vi "remote_I(t)-T at fixed V (V recorded), Ver. 2.vi"() -> ()   [LabVIEW 2014]
uses:
  C:/Program Files (x86)/National Instruments/LabVIEW 2014/examples/Instrument IO/Serial/support/Serial - Settings.ctl
  <vilib>/Instr/_visa.llb/VISA Configure Serial Port (Instr).vi
panel:
  out "Start":bool
  in  "获取的数据的字节最大值":u32=1000
  in  "终止符":u8=10 format="%.0x"
  in  "COM":refnum<visa-resource-name>="COM5"
  in  "串口设置":T1={"波特率"=38400, "数据比特"=8, "奇偶"=enum."None", "停止位"=10, "流控制"=0} {"流控制" items=["无"=0, "XON/XOFF"=1, "RTS/CTS"=2, "DTR/DSR"=4]; "停止位" items=["1.0"=10, "1.5"=15, "2.0"=20]; "数据比特" min=5 max=8 step=1; "波特率" items=["75"=75, "110"=110, "134"=134, "150"=150, "300"=300, "600"=600, "1200"=1200, "1800"=1800, "2400"=2400, "4800"=4800, "7200"=7200, "9600"=9600, "14400"=14400, "19200"=19200, "28800"=28800, "38400"=38400, "56000"=56000, "57600"=57600, "115200"=115200, "128000"=128000, "230400"=230400]}
  in  "终止符时结束读取？":bool=TRUE
  in  "Compliance":sgl=50.0
  in  "Start":bool
  out "File Path":path
  in  "Negative t":u32
  in  "Positive t":u32
  in  "Negative V":dbl min=-3.0 max=0.0
  in  "Positive V":dbl min=0.0 max=5.0 format="%#_3g"
  out "XY Graph":cluster{dbl[], dbl[]}[](graph)
  # "s"
  # "s"
  # "mA"
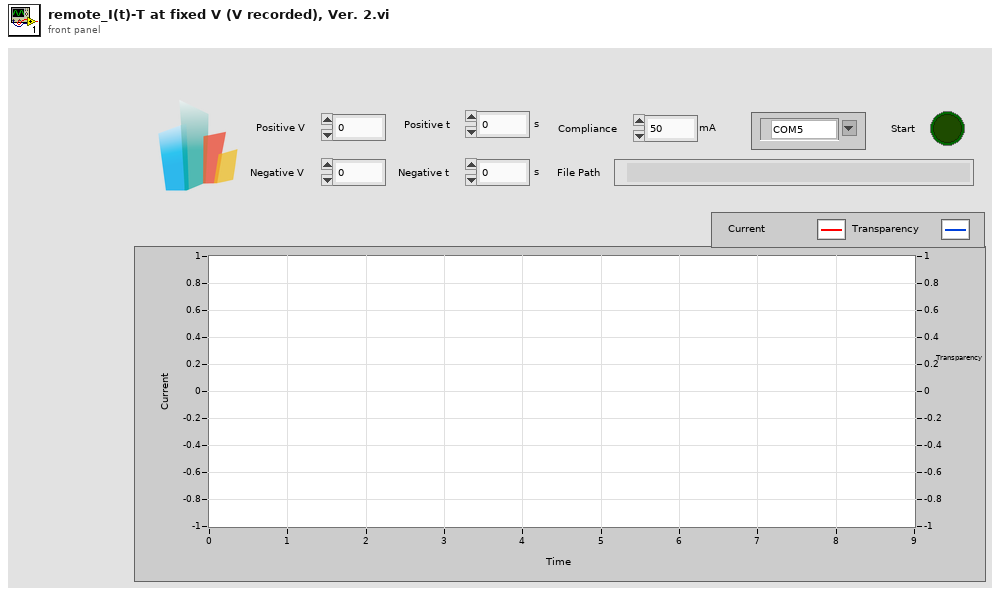
[diagram p1: front panel]
types:
  T1 = typedef "Serial - Settings.ctl" = cluster{"波特率":u32, "数据比特":u16, "奇偶":enum16{"None", "Odd", "Even", "Mark", "Space"}, "停止位":u16, "流控制":u16}
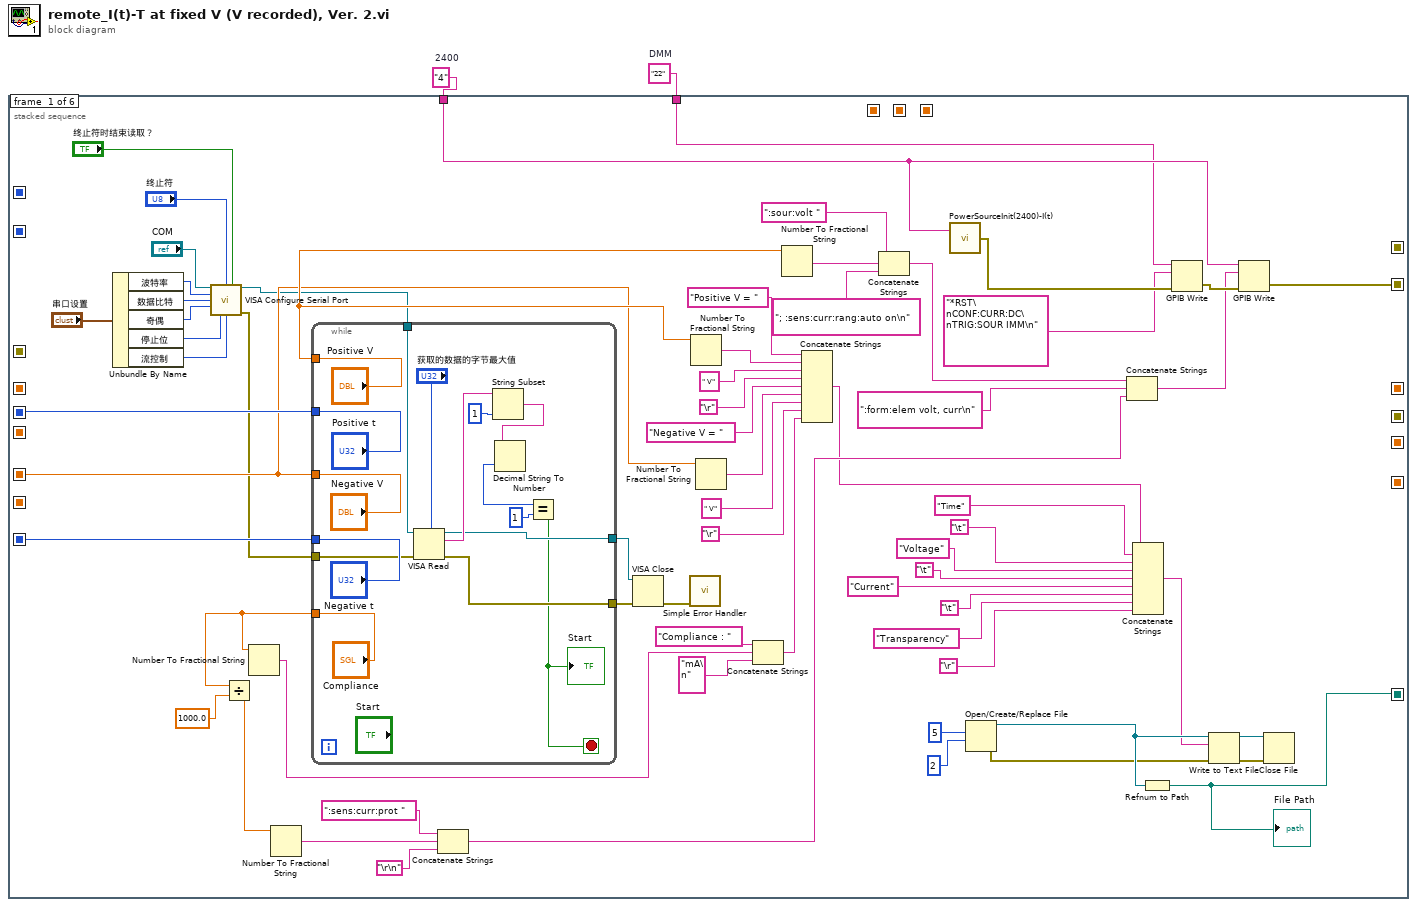
[diagram p0: block diagram]
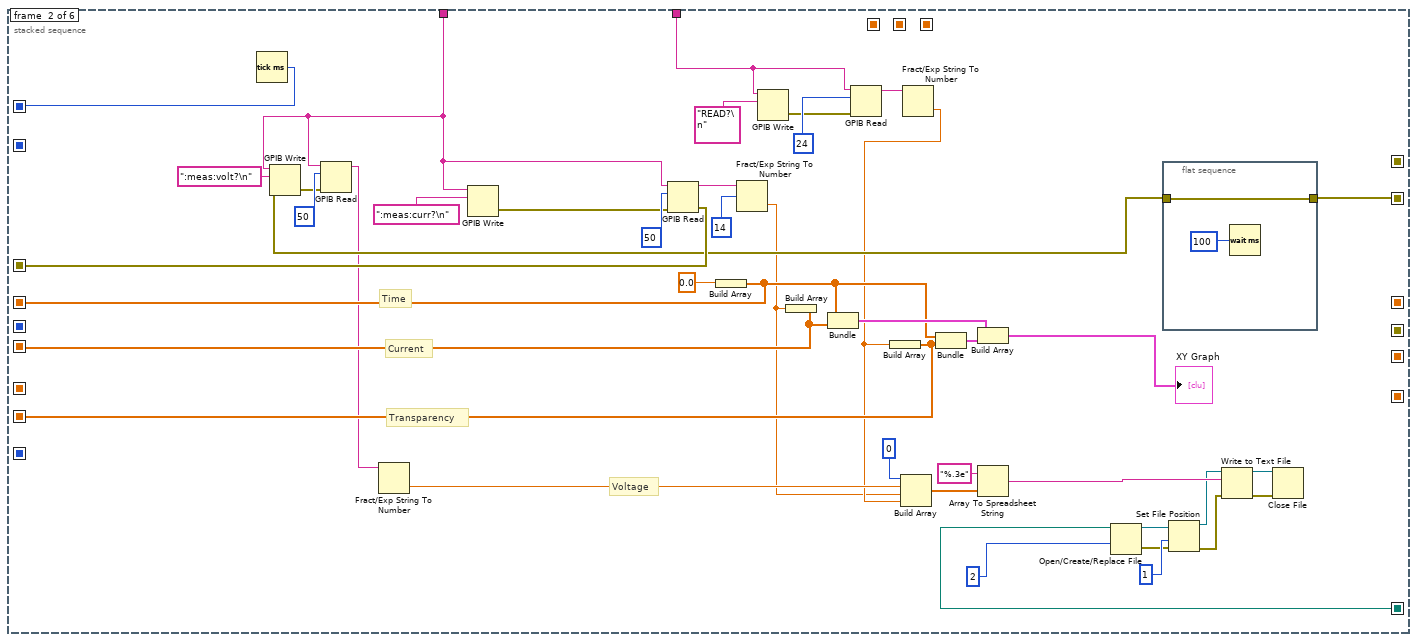
[diagram p2: hidden frame]
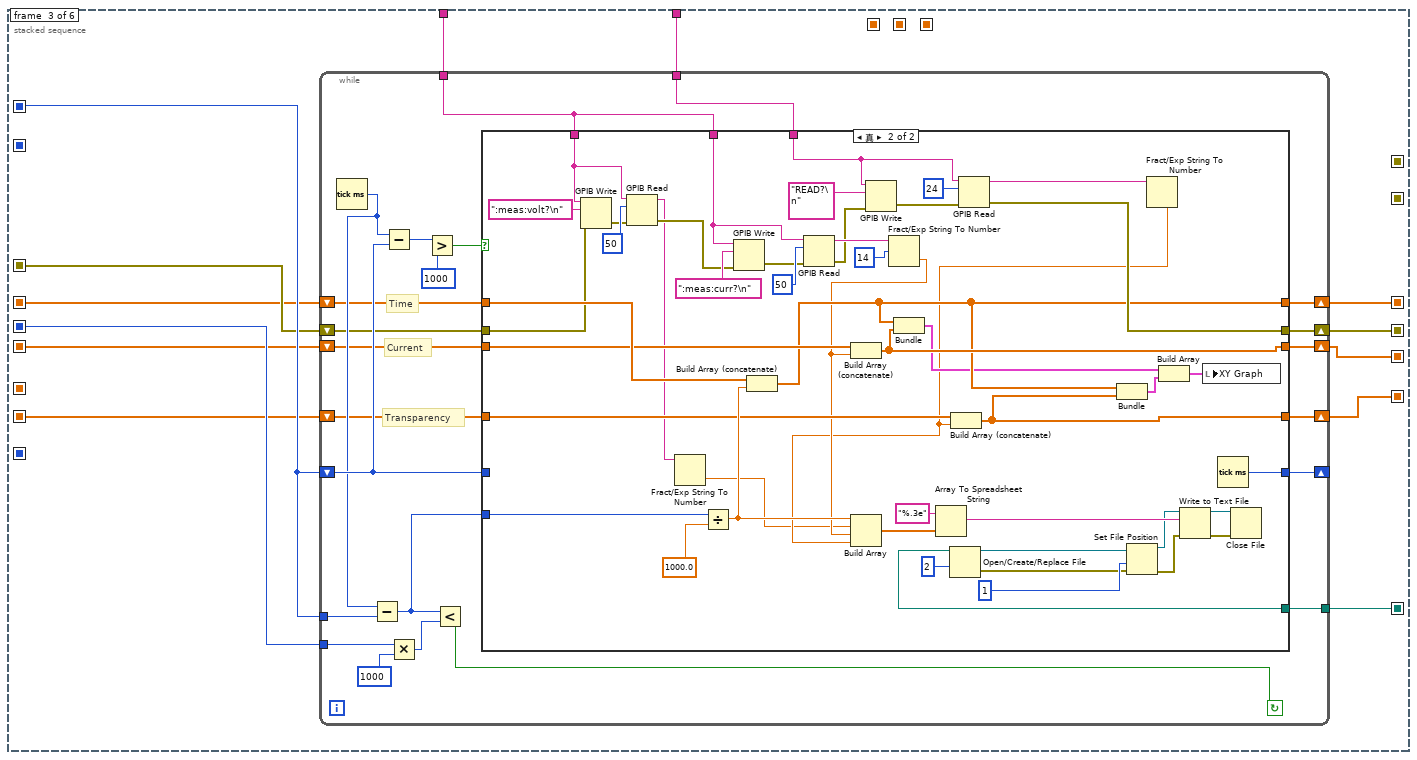
[diagram p3: hidden frame]
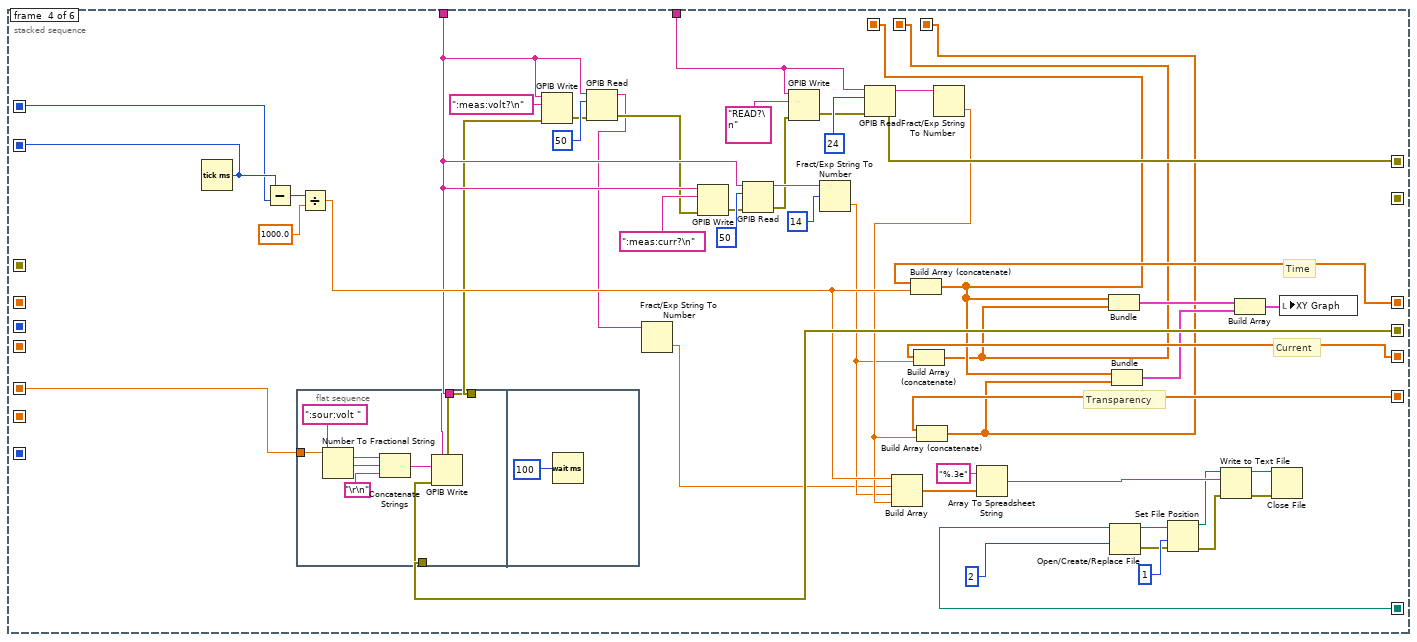
[diagram p5: hidden frame]
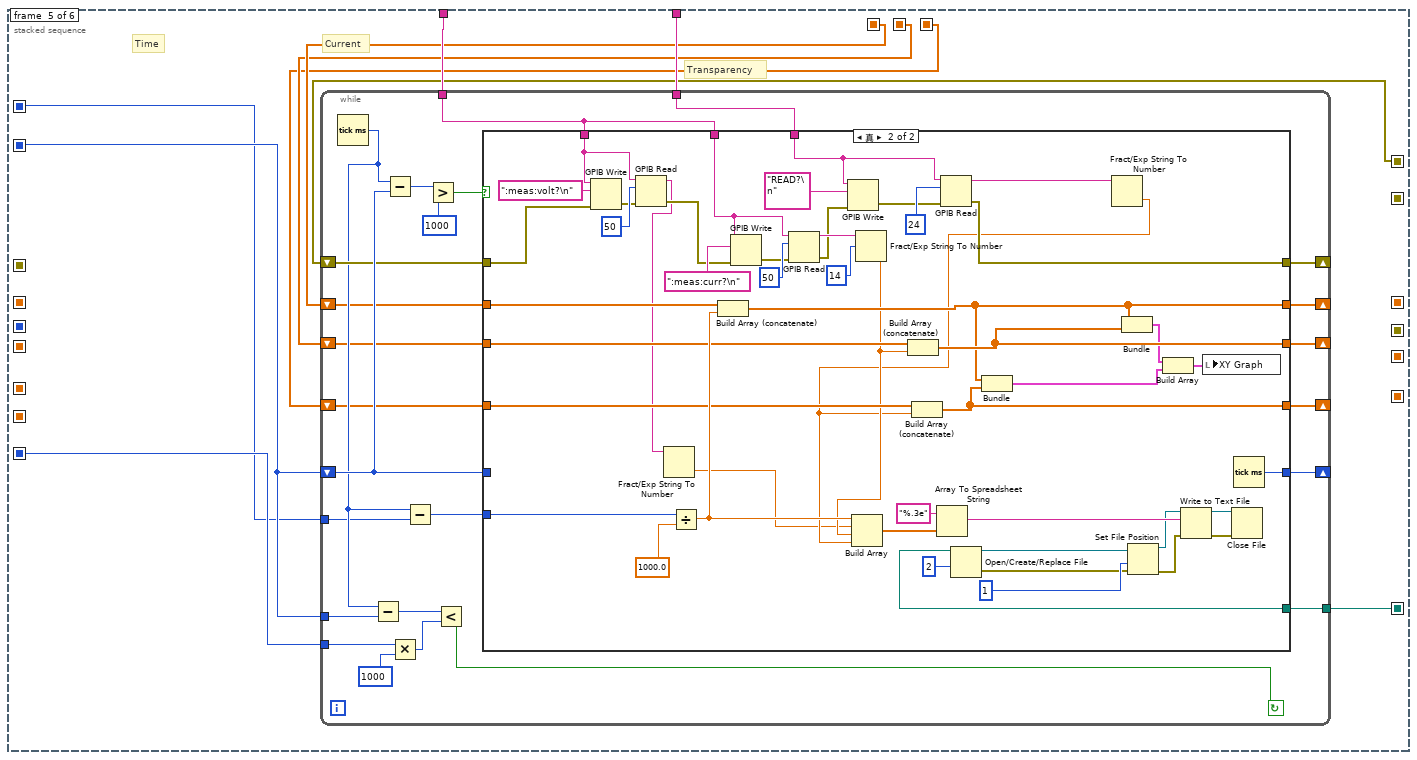
[diagram p6: hidden frame]
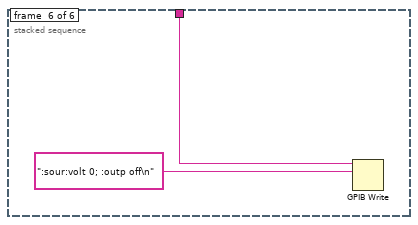
[diagram p8: hidden frame]
diagram:
  w2 = "4"  # 2400
  w1 = "22"  # DMM
  n1 = stacked-sequence {
    seq-local: [w41 _ _ _ _ _] -> [_ _ w141 _ _ _]
    seq-local: [w40 _ _ _ _ _] -> [_ w122 _ _ _ _]
    seq-local: [w39 _ _ _ _ _] -> [_ w104 w137 w246 w284 _]
    seq-local: [_ w103 _ _ _ _] -> [_ _ w140 w239 w280 _]
    seq-local: [_ w102 _ _ _ _] -> [_ _ w136 _ _ _]
    seq-local: [_ _ w135 _ _ _] -> [_ _ _ w244 _ _]
    seq-local: [w38 _ _ _ _ _] -> [_ _ _ w247 _ _]
    seq-local: [w37 _ _ _ _ _] -> [_ _ _ _ w282 _]
    seq-local: [_ _ w134 _ _ _] -> [_ _ _ w236 _ _]
    seq-local: [_ _ _ w243 _ _] -> [_ _ _ _ w283 _]
    seq-local: [_ _ _ w240 _ _] -> [_ _ _ _ w281 _]
    seq-local: [_ w97 _ _ _ _] -> [_ _ w133 _ _ _]
    seq-local: [_ w96 _ _ _ _] -> [_ _ w132 _ _ _]
    seq-local: [_ w95 _ _ _ _] -> [_ _ w131 _ _ _]
    seq-local: [_ _ w130 _ _ _] -> [_ _ _ w238 _ _]
    seq-local: [_ _ w129 _ _ _] -> [_ _ _ w237 _ _]
    seq-local: [_ _ _ w232 _ _] -> [_ _ _ _ w279 _]
    seq-local: [_ _ _ w231 _ _] -> [_ _ _ _ w278 _]
    seq-local: [_ _ _ w230 _ _] -> [_ _ _ _ w277 _]
    tunnel: w2 -> [w43 w85 w139 w224 w286 w365]
    tunnel: w1 -> [w42 w106 w138 w248 w285 _]
    frame #0 {
      n2 = Unbundle By Name("串口设置") -> ("波特率"=w12:u32, "数据比特"=w13:u16, "奇偶"=w14:enum16{"None", "Odd", "Even", "Mark", "Space"}, "停止位"=w15:u16, "流控制"=w9:u16)
      n3 = call-poly "VISA Configure Serial Port"("VISA resource name"="COM", "termination char\n(0xA = '\\n' = LF)"="终止符", "Enable Termination\nChar (T)"="终止符时结束读取？", "baud rate (9600)"=w12, "data bits (8)"=w13, "parity (0:none)"=w14, "stop bits (10: 1 bit)"=w15, "flow control (0:none)"=w9) -> ("VISA resource name out"=w4:refnum<visa-resource-name>, "error out"=w3:errorcluster)  [unwired: 2 in, 4 out]
      n4 = while {
        tunnel: ["Positive V"] -> w46
        tunnel: ["Positive t"] -> w41
        tunnel: ["Negative V"] -> w38
        tunnel: ["Negative t"] -> w37
        tunnel: ["Compliance"] -> w31
        tunnel: [w73] -> w6
        tunnel: [w72] -> w5
        tunnel: w4 -> [w71]
        tunnel: w3 -> [w70]
        stop <- w69 stop-if-true
        n5 = VISA Read(VISA resource name=w71, byte count="获取的数据的字节最大值", error in (no error)=w70) -> (VISA resource name out=w72:refnum<visa-resource-name>, read buffer=w75:string, error out=w73:errorcluster)  [unwired: 1 out]
        n6 = String Subset(string=w75, length (rest)=1 ("长度（剩余）")) -> (substring=w77:string)  [unwired: 1 in]
        n7 = Decimal String To Number(string=w77) -> (number=w78:i32)  [unwired: 2 in, 1 out]
        n8 = Equal?(x=w78, y=1) -> (x = y?=w69:bool)
        "Start" <- w69
      }
      n9 = Divide(x=w31, y=1000.0) -> (x/y=w30:dbl)
      n10 = Number To Fractional String(number=w31) -> (F-format string=w27:string)  [unwired: 3 in]
      n11 = Number To Fractional String(number=w30) -> (F-format string=w34:string)  [unwired: 3 in]
      n12 = Concatenate Strings(":sens:curr:prot ", w34, "\r\n") -> (w23:string)
      n13 = VISA Close(VISA resource name=w5, error in (no error)=w6) -> (error out=w7:errorcluster)
      n14 = call <vilib>:"Simple Error Handler.vi"("error in (no error)"=w7) -> ()  [unwired: 1 in, 8 out]
      n15 = Number To Fractional String(number=w46) -> (F-format string=w55:string)  [unwired: 3 in]
      n16 = Number To Fractional String(number=w38) -> (F-format string=w51:string)  [unwired: 3 in]
      n17 = Concatenate Strings("Compliance : ", w27, "mA\n") -> (w26:string)
      n18 = Number To Fractional String(number=w46) -> (F-format string=w47:string)  [unwired: 3 in]
      n19 = Concatenate Strings("Positive V = ", w55, " V", "\r", "Negative V = ", w51, " V", "\r", w26) -> (w21:string)
      n20 = Concatenate Strings(":sour:volt ", w47, "; :sens:curr:rang:auto on\n") -> (w25:string)
      n21 = call "PowerSourceInit(2400)-I(t).vi"("K2400 Address"=w43) -> ("error out"=w67:errorcluster)  [unwired: 1 in]
      n22 = Open/Create/Replace File(operation (0:open)=5, access (0:read/write)=2) -> (refnum out=w62:refnum<file>, error out=w59:errorcluster)  [unwired: 4 in, 1 out]
      n23 = Concatenate Strings(w25, ":form:elem volt, curr\n", w23) -> (w24:string)
      n24 = Concatenate Strings(w21, "Time", "\t", "Voltage", "\t", "Current", "\t", "Transparency", "\r") -> (w61:string)
      n25 = Refnum to Path(1:w62) -> (0:w39:path)
      "File Path" <- w39
      n26 = GPIB Write(0:w42, 1:"*RST\nCONF:CURR:DC\nTRIG:SOUR IMM\n", 3:w67) -> (6:w44:errorcluster)  [unwired: 2 in, 1 out]
      n27 = Write to Text File(file (use dialog)=w62, text=w61, error in=w59) -> (refnum out=w58:refnum<file>, error out=w60:errorcluster)  [unwired: 1 in, 1 out]
      n28 = GPIB Write(0:w43, 1:w24, 3:w44) -> (6:w40:errorcluster)  [unwired: 2 in, 1 out]
      n29 = Close File(refnum=w58, error in=w60) -> ()  [unwired: 2 out]
    }
    frame #1 {
      # "Voltage"
      # "Transparency"
      # "Current"
      # "Time"
      n30 = Tick Count (ms)() -> (millisecond timer value=w103:u32)
      n31 = GPIB Write(0:w85, 1:":meas:volt?\n", 3:w91) -> (6:w93:errorcluster)  [unwired: 2 in, 1 out]
      n32 = GPIB Read(0:w85, 1:50, 3:w93) -> (5:w90:string)  [unwired: 2 in, 2 out]
      n33 = Fract/Exp String To Number(string=w90) -> (number=w89:dbl)  [unwired: 3 in, 1 out]
      n34 = GPIB Write(0:w85, 1:":meas:curr?\n") -> (6:w124:errorcluster)  [unwired: 3 in, 1 out]
      n35 = GPIB Read(0:w85, 1:50, 3:w124) -> (5:w125:string, 7:w102:errorcluster)  [unwired: 2 in, 1 out]
      n36 = Build Array(0.0) -> (w97:dbl[])
      n37 = Fract/Exp String To Number(string=w125, offset=14) -> (number=w87:dbl)  [unwired: 2 in, 1 out]
      n38 = GPIB Write(0:w106, 1:"READ?\n") -> (6:w108:errorcluster)  [unwired: 3 in, 1 out]
      n39 = Build Array(w87) -> (w96:dbl[])
      n40 = Bundle(w97, w96) -> (w99:cluster{dbl[], dbl[]})  [unwired: 1 in]
      n41 = GPIB Read(0:w106, 1:24, 3:w108) -> (5:w107:string)  [unwired: 2 in, 2 out]
      n42 = Fract/Exp String To Number(string=w107) -> (number=w88:dbl)  [unwired: 3 in, 1 out]
      n43 = Build Array(w88) -> (w95:dbl[])
      n44 = Build Array(0, w89, w87, w88) -> (w120:dbl[])
      n45 = Bundle(w97, w95) -> (w100:cluster{dbl[], dbl[]})  [unwired: 1 in]
      n46 = Build Array(w99, w100) -> (→"XY Graph":cluster{dbl[], dbl[]}[])
      n47 = Array To Spreadsheet String(array=w120, 3:"%.3e") -> (spreadsheet string=w118:string)  [unwired: 1 out]
      n48 = Open/Create/Replace File(file path (use dialog)=w104, access (0:read/write)=2) -> (refnum out=w115:refnum<file>, error out=w113:errorcluster)  [unwired: 4 in, 1 out]
      n49 = flat-sequence {
        tunnel: [w127] -> w91
        tunnel: w122 -> [w127]
        frame #0 {
          n50 = Wait (ms)(milliseconds to wait=100) -> ()  [unwired: 1 out]
        }
      }
      n51 = Set File Position(refnum=w115, from (0:start)=1, error in=w113) -> (refnum out=w112:refnum<file>, error out=w111:errorcluster)  [unwired: 1 in]
      n52 = Write to Text File(file (use dialog)=w112, text=w118, error in=w111) -> (refnum out=w116:refnum<file>, error out=w117:errorcluster)  [unwired: 1 in, 1 out]
      n53 = Close File(refnum=w116, error in=w117) -> ()  [unwired: 2 out]
    }
    frame #2 {
      n54 = while {
        shift-right: [w161] -> _
        shift-left: w140 -> [w160]
        tunnel: w140 -> [w158]
        tunnel: w141 -> [w157]
        tunnel: w139 -> [w142]
        tunnel: w138 -> [w153]
        tunnel: w137 -> [w152]
        shift-right: [w149] -> w135
        shift-left: w136 -> [w150]
        shift-right: [w143] -> w134
        shift-left: w131 -> [w144]
        shift-right: [w146] -> w130
        shift-left: w133 -> [w148]
        shift-right: [w145] -> w129
        shift-left: w132 -> [w147]
        stop <- w154 continue-if-true
        # "Transparency"
        # "Current"
        # "Time"
        n55 = Tick Count (ms)() -> (millisecond timer value=w159:u32)
        n56 = Subtract(x=w159, y=w158) -> (x-y=w151:u32)
        n57 = Subtract(x=w159, y=w160) -> (x-y=w164:u32)
        n58 = Multiply(x=w157, y=1000) -> (x*y=w155:u32)
        n59 = Greater?(x=w164, y=1000) -> (0:w162:bool)
        n60 = Less?(x=w151, y=w155) -> (x < y?=w154:bool)
        n61 = case shown="真" w162 {
          tunnel: [w169 w217] -> w161
          tunnel: w160 -> [w169 _]
          tunnel: w142 -> [_ w208]
          tunnel: w153 -> [_ w207]
          tunnel: w152 -> [_ w195]
          tunnel: w151 -> [_ w193]
          tunnel: w150 -> [w168 w176]
          tunnel: [w168 w191] -> w149
          tunnel: w148 -> [w167 w190]
          tunnel: w147 -> [w166 w188]
          tunnel: [w167 w185] -> w146
          tunnel: [w166 w186] -> w145
          tunnel: w144 -> [w165 w187]
          tunnel: [w165 w184] -> w143
          tunnel: w142 -> [_ w177]
          frame False {
          }
          frame True {
            n62 = GPIB Write(0:w177, 1:":meas:volt?\n", 3:w176) -> (6:w179:errorcluster)  [unwired: 2 in, 1 out]
            n63 = GPIB Read(0:w177, 1:50, 3:w179) -> (5:w173:string, 7:w175:errorcluster)  [unwired: 2 in, 1 out]
            n64 = Fract/Exp String To Number(string=w173) -> (number=w170:dbl)  [unwired: 3 in, 1 out]
            n65 = Divide(x=w193, y=1000.0) -> (x/y=w189:dbl)
            n66 = GPIB Write(0:w208, 1:":meas:curr?\n", 3:w175) -> (6:w214:errorcluster)  [unwired: 2 in, 1 out]
            n67 = Build Array (concatenate)(w190, w189) -> (w185:dbl[])
            n68 = GPIB Read(0:w208, 1:50, 3:w214) -> (5:w215:string, 7:w192:errorcluster)  [unwired: 2 in, 1 out]
            n69 = GPIB Write(0:w207, 1:"READ?\n", 3:w192) -> (6:w210:errorcluster)  [unwired: 2 in, 1 out]
            n70 = Fract/Exp String To Number(string=w215, offset=14) -> (number=w172:dbl)  [unwired: 2 in, 1 out]
            n71 = Build Array (concatenate)(w188, w172) -> (w186:dbl[])
            n72 = Bundle(w185, w186) -> (w183:cluster{dbl[], dbl[]})  [unwired: 1 in]
            n73 = Open/Create/Replace File(file path (use dialog)=w195, access (0:read/write)=2) -> (refnum out=w200:refnum<file>, error out=w198:errorcluster)  [unwired: 4 in, 1 out]
            n74 = GPIB Read(0:w207, 1:24, 3:w210) -> (5:w209:string, 7:w191:errorcluster)  [unwired: 2 in, 1 out]
            n75 = Set File Position(refnum=w200, from (0:start)=1, error in=w198) -> (refnum out=w197:refnum<file>, error out=w196:errorcluster)  [unwired: 1 in]
            n76 = Fract/Exp String To Number(string=w209) -> (number=w171:dbl)  [unwired: 3 in, 1 out]
            n77 = Build Array(w189, w170, w172, w171) -> (w205:dbl[])
            n78 = Array To Spreadsheet String(array=w205, 3:"%.3e") -> (spreadsheet string=w203:string)  [unwired: 1 out]
            n79 = Build Array (concatenate)(w187, w171) -> (w184:dbl[])
            n80 = Bundle(w185, w184) -> (w182:cluster{dbl[], dbl[]})  [unwired: 1 in]
            n81 = Build Array(w183, w182) -> (w181:cluster{dbl[], dbl[]}[])
            n82 = Write to Text File(file (use dialog)=w197, text=w203, error in=w196) -> (refnum out=w201:refnum<file>, error out=w202:errorcluster)  [unwired: 1 in, 1 out]
            n83 = local write "XY Graph"(w181) -> ()
            n84 = Tick Count (ms)() -> (millisecond timer value=w217:u32)
            n85 = Close File(refnum=w201, error in=w202) -> ()  [unwired: 2 out]
          }
        }
      }
    }
    frame #3 {
      # "Transparency"
      # "Current"
      # "Time"
      n86 = Tick Count (ms)() -> (millisecond timer value=w240:u32)
      n87 = Subtract(x=w240, y=w239) -> (x-y=w242:u32)
      n88 = flat-sequence {
        tunnel: w247 -> [w272]
        tunnel: w224 -> [w270]
        tunnel: [w269] -> w223
        tunnel: w244 -> [w268]
        frame #0 {
          n89 = Number To Fractional String(number=w272) -> (F-format string=w274:string)  [unwired: 3 in]
          n90 = Concatenate Strings(":sour:volt ", w274, "\r\n") -> (w271:string)
          n91 = GPIB Write(0:w270, 1:w271, 3:w268) -> (6:w269:errorcluster)  [unwired: 2 in, 1 out]
        }
        frame #1 {
          n92 = Wait (ms)(milliseconds to wait=100) -> ()  [unwired: 1 out]
        }
      }
      n93 = Divide(x=w242, y=1000.0) -> (x/y=w229:dbl)
      n94 = GPIB Write(0:w224, 1:":meas:volt?\n", 3:w223) -> (6:w226:errorcluster)  [unwired: 2 in, 1 out]
      n95 = GPIB Read(0:w224, 1:50, 3:w226) -> (5:w221:string, 7:w222:errorcluster)  [unwired: 2 in, 1 out]
      n96 = Fract/Exp String To Number(string=w221) -> (number=w218:dbl)  [unwired: 3 in, 1 out]
      n97 = GPIB Write(0:w224, 1:":meas:curr?\n", 3:w222) -> (6:w265:errorcluster)  [unwired: 2 in, 1 out]
      n98 = GPIB Read(0:w224, 1:50, 3:w265) -> (5:w266:string, 7:w245:errorcluster)  [unwired: 2 in, 1 out]
      n99 = GPIB Write(0:w248, 1:"READ?\n", 3:w245) -> (6:w250:errorcluster)  [unwired: 2 in, 1 out]
      n100 = Fract/Exp String To Number(string=w266, offset=14) -> (number=w219:dbl)  [unwired: 2 in, 1 out]
      n101 = GPIB Read(0:w248, 1:24, 3:w250) -> (5:w249:string, 7:w243:errorcluster)  [unwired: 2 in, 1 out]
      n102 = Build Array (concatenate)(w238, w229) -> (w232:dbl[])
      n103 = Build Array (concatenate)(w237, w219) -> (w231:dbl[])
      n104 = Fract/Exp String To Number(string=w249) -> (number=w220:dbl)  [unwired: 3 in, 1 out]
      n105 = Build Array(w229, w218, w219, w220) -> (w262:dbl[])
      n106 = Build Array (concatenate)(w236, w220) -> (w230:dbl[])
      n107 = Array To Spreadsheet String(array=w262, 3:"%.3e") -> (spreadsheet string=w260:string)  [unwired: 1 out]
      n108 = Bundle(w232, w231) -> (w235:cluster{dbl[], dbl[]})  [unwired: 1 in]
      n109 = Open/Create/Replace File(file path (use dialog)=w246, access (0:read/write)=2) -> (refnum out=w257:refnum<file>, error out=w255:errorcluster)  [unwired: 4 in, 1 out]
      n110 = Bundle(w232, w230) -> (w234:cluster{dbl[], dbl[]})  [unwired: 1 in]
      n111 = Set File Position(refnum=w257, from (0:start)=1, error in=w255) -> (refnum out=w254:refnum<file>, error out=w253:errorcluster)  [unwired: 1 in]
      n112 = Write to Text File(file (use dialog)=w254, text=w260, error in=w253) -> (refnum out=w258:refnum<file>, error out=w259:errorcluster)  [unwired: 1 in, 1 out]
      n113 = Build Array(w235, w234) -> (w233:cluster{dbl[], dbl[]}[])
      n114 = Close File(refnum=w258, error in=w259) -> ()  [unwired: 2 out]
      n115 = local write "XY Graph"(w233) -> ()
    }
    frame #4 {
      # "Transparency"
      # "Current"
      # "Time"
      n116 = while {
        shift-right: [w308] -> _
        shift-left: w281 -> [w307]
        tunnel: w281 -> [w306]
        tunnel: w282 -> [w305]
        tunnel: w286 -> [w287]
        tunnel: w285 -> [w301]
        tunnel: w284 -> [w300]
        shift-right: [w297] -> _
        shift-left: w283 -> [w298]
        shift-right: [w290] -> _
        shift-left: w278 -> [w291]
        tunnel: w280 -> [w294]
        shift-right: [w292] -> _
        shift-left: w279 -> [w293]
        shift-right: [w288] -> _
        shift-left: w277 -> [w289]
        stop <- w302 continue-if-true
        n117 = Tick Count (ms)() -> (millisecond timer value=w295:u32)
        n118 = Subtract(x=w295, y=w306) -> (x-y=w299:u32)
        n119 = Subtract(x=w295, y=w307) -> (x-y=w311:u32)
        n120 = Multiply(x=w305, y=1000) -> (x*y=w303:u32)
        n121 = Subtract(x=w295, y=w294) -> (x-y=w296:u32)
        n122 = Greater?(x=w311, y=1000) -> (0:w309:bool)
        n123 = Less?(x=w299, y=w303) -> (x < y?=w302:bool)
        n124 = case shown="真" w309 {
          tunnel: [w316 w364] -> w308
          tunnel: w307 -> [w316 _]
          tunnel: w287 -> [_ w355]
          tunnel: w301 -> [_ w354]
          tunnel: w300 -> [_ w342]
          tunnel: w296 -> [_ w340]
          tunnel: w298 -> [w315 w322]
          tunnel: [w315 w338] -> w297
          tunnel: w293 -> [w314 w337]
          tunnel: [w314 w331] -> w292
          tunnel: w291 -> [w313 w335]
          tunnel: [w313 w334] -> w290
          tunnel: w289 -> [w312 w333]
          tunnel: [w312 w332] -> w288
          tunnel: w287 -> [_ w323]
          frame False {
          }
          frame True {
            n125 = GPIB Write(0:w323, 1:":meas:volt?\n", 3:w322) -> (6:w325:errorcluster)  [unwired: 2 in, 1 out]
            n126 = GPIB Read(0:w323, 1:50, 3:w325) -> (5:w320:string, 7:w321:errorcluster)  [unwired: 2 in, 1 out]
            n127 = Fract/Exp String To Number(string=w320) -> (number=w317:dbl)  [unwired: 3 in, 1 out]
            n128 = Divide(x=w340, y=1000.0) -> (x/y=w336:dbl)
            n129 = Build Array (concatenate)(w337, w336) -> (w331:dbl[])
            n130 = GPIB Write(0:w355, 1:":meas:curr?\n", 3:w321) -> (6:w361:errorcluster)  [unwired: 2 in, 1 out]
            n131 = GPIB Read(0:w355, 1:50, 3:w361) -> (5:w362:string, 7:w339:errorcluster)  [unwired: 2 in, 1 out]
            n132 = GPIB Write(0:w354, 1:"READ?\n", 3:w339) -> (6:w357:errorcluster)  [unwired: 2 in, 1 out]
            n133 = Fract/Exp String To Number(string=w362, offset=14) -> (number=w319:dbl)  [unwired: 2 in, 1 out]
            n134 = Build Array (concatenate)(w335, w319) -> (w334:dbl[])
            n135 = GPIB Read(0:w354, 1:24, 3:w357) -> (5:w356:string, 7:w338:errorcluster)  [unwired: 2 in, 1 out]
            n136 = Open/Create/Replace File(file path (use dialog)=w342, access (0:read/write)=2) -> (refnum out=w347:refnum<file>, error out=w345:errorcluster)  [unwired: 4 in, 1 out]
            n137 = Fract/Exp String To Number(string=w356) -> (number=w318:dbl)  [unwired: 3 in, 1 out]
            n138 = Build Array(w336, w317, w319, w318) -> (w352:dbl[])
            n139 = Build Array (concatenate)(w333, w318) -> (w332:dbl[])
            n140 = Array To Spreadsheet String(array=w352, 3:"%.3e") -> (spreadsheet string=w350:string)  [unwired: 1 out]
            n141 = Bundle(w331, w332) -> (w329:cluster{dbl[], dbl[]})  [unwired: 1 in]
            n142 = Bundle(w331, w334) -> (w330:cluster{dbl[], dbl[]})  [unwired: 1 in]
            n143 = Set File Position(refnum=w347, from (0:start)=1, error in=w345) -> (refnum out=w344:refnum<file>, error out=w343:errorcluster)  [unwired: 1 in]
            n144 = Build Array(w330, w329) -> (w328:cluster{dbl[], dbl[]}[])
            n145 = Write to Text File(file (use dialog)=w344, text=w350, error in=w343) -> (refnum out=w348:refnum<file>, error out=w349:errorcluster)  [unwired: 1 in, 1 out]
            n146 = local write "XY Graph"(w328) -> ()
            n147 = Close File(refnum=w348, error in=w349) -> ()  [unwired: 2 out]
            n148 = Tick Count (ms)() -> (millisecond timer value=w364:u32)
          }
        }
      }
    }
    frame #5 {
      n149 = GPIB Write(0:w365, 1:":sour:volt 0; :outp off\n") -> ()  [unwired: 3 in, 2 out]
    }
  }
